vi "gentec-SOLO-PE.Current Measurement.vi"(8 "error in (no error)":errorcluster, 11 "VISA Refnum in":refnum<visa-resource-name>) -> (0 "error out":errorcluster, 1 "Uncorrected Value [J]":dbl, 2 "Error":string, 3 "VISA Refnum out":refnum<visa-resource-name>, 4 "Timeout":bool, 6 "Corrected Value [J]":dbl)   [LabVIEW 2014, in "gentec-SOLO-PE - Driver.lvlib"]
doc: "This VI reads out the current value. The uncorrected is the raw value while the corrected value is corrcted by a multiplier and an offset."
uses:
  gentec-SOLO-PE - Driver.lvlib
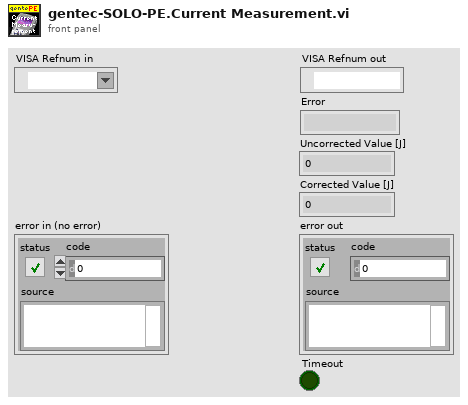
[diagram p1: front panel]
types:
  T1 = cluster{"Return Parameters[0]":u32, "Return Parameters[1]":u32, "Return Parameters[2]":u32, "Return Parameters[3]":u32}
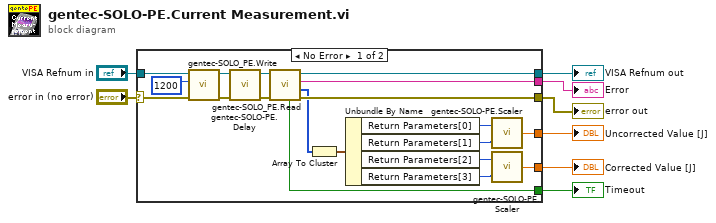
[diagram p0: block diagram]
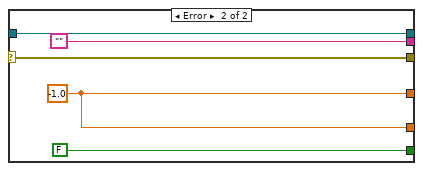
[diagram p2: hidden frame]
diagram:
  n1 = case shown="No Error" "error in (no error)" {
    selector: "error in (no error)" -> [w19 w31]
    tunnel: [w17 w31] -> w8
    tunnel: [w27 w32] -> w7
    tunnel: [w18 ""] -> w3
    tunnel: [w26 FALSE ("Timeout")] -> w6
    tunnel: "VISA Refnum in" -> [w21 w32]
    tunnel: [w10 w28] -> w2
    tunnel: [w9 w28] -> w1
    frame No Error {
      n2 = call "gentec-SOLO_PE.Write.vi"("error in (no error)"=w19, "Command Handle"=u16 1200, "VISA Refnum in"=w21) -> ("error out"=w24:errorcluster, "VISA Refnum out"=w22:refnum<visa-resource-name>)  [unwired: 7 in]
      n3 = call "gentec-SOLO-PE.Delay.vi"("error in (no error)"=w24, "VISA resource In"=w22) -> ("error out"=w25:errorcluster, "VISA resource Out"=w23:refnum<visa-resource-name>)  [unwired: 4 in]
      n4 = call "gentec-SOLO_PE.Read.vi"("error in (no error)"=w25, "VISA Refnum in"=w23) -> ("error out"=w17:errorcluster, "Return Parameters"=w11:u32[], "Error"=w18:string, "VISA Refnum out"=w27:refnum<visa-resource-name>, "Timeout"=w26:bool)  [unwired: 5 in]
      n5 = Array To Cluster(array=w11) -> (cluster=w16:T1)
      n6 = Unbundle By Name(w16) -> ("Return Parameters[0]"=w15:u32, "Return Parameters[1]"=w14:u32, "Return Parameters[2]"=w12:u32, "Return Parameters[3]"=w13:u32)
      n7 = call "gentec-SOLO-PE.Scaler.vi"("Scaler"=w14, "Value"=w15) -> ("Scaled Value"=w10:dbl)
      n8 = call "gentec-SOLO-PE.Scaler.vi"("Scaler"=w13, "Value"=w12) -> ("Scaled Value"=w9:dbl)
    }
    frame Error {
      w28 = -1.0 ("Scaled Value")
    }
  }
  "error out" <- w8
  "VISA Refnum out" <- w7
  "Error" <- w3
  "Timeout" <- w6
  "Uncorrected Value [J]" <- w2
  "Corrected Value [J]" <- w1
